vi "Test Remove From Child List.vi"(8 "error in (no error)":errorcluster) -> (0 "error out":errorcluster)   [LabVIEW 2017, in "Unit Tests.lvlib"]
uses:
  Unit Tests.lvlib
  source/Browser Core/Node Classes/Generic Node/Generic Node.lvclass
  source/Browser Core/Node Classes/Generic Node/Generic Node.lvclass/Generic Node.ctl
  <vilib>/addons/_JKI Toolkits/Caraya/classes/Test/Test.lvclass
  <vilib>/addons/_JKI Toolkits/Caraya/classes/Assert/Assert.lvclass
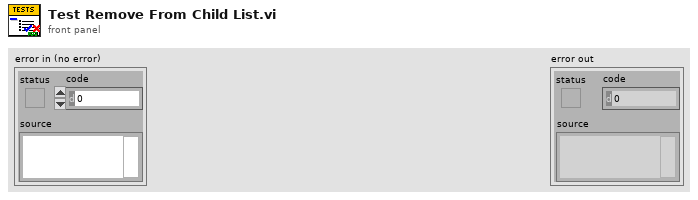
[diagram p1: front panel]
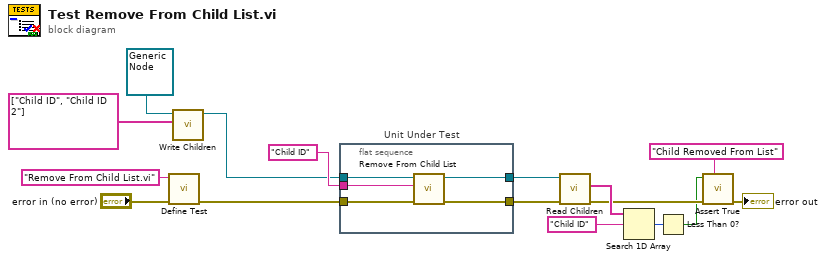
[diagram p0: block diagram]
diagram:
  n1 = call <vilib>:"Define Test.vi"("error in (no error)"="error in (no error)", "Label (VI Title)"="Remove From Child List.vi") -> ("error out"=w10:errorcluster)  [unwired: 9 in]
  n2 = call "Write Children.vi"("Children"=string[] ["Child ID", "Child ID 2"], "Generic Node in"=refnum<class "Generic Node.lvclass"> refnum) -> ("Generic Node out"=w12:refnum<class "Generic Node.lvclass">)  [unwired: 8 in, 1 out]
  n3 = flat-sequence "Unit Under Test" {
    tunnel: w12 -> [w21]
    tunnel: "Child ID" ("Child ID") -> [w20]
    tunnel: w10 -> [w19]
    tunnel: [w18] -> w9
    tunnel: [w17] -> w8
    frame #0 {
      n4 = call "Remove From Child List.vi"("error in (no error)"=w19, "Child ID"=w20, "Generic Node in"=w21) -> ("error out"=w18:errorcluster, "Generic Node out"=w17:refnum<class "Generic Node.lvclass">)  [unwired: 7 in]
    }
  }
  n5 = call "Read Children.vi"("error in (no error)"=w9, "Generic Node in"=w8) -> ("error out"=w4:errorcluster, "Children"=w7:string[])  [unwired: 7 in, 1 out]
  n6 = Search 1D Array(1D array=w7, element="Child ID" ("UID")) -> (index of element=w5:i32)  [unwired: 1 in]
  n7 = Less Than 0?(x=w5) -> (x < 0?=w3:bool)
  n8 = call <vilib>:"Assert True.vi"("Label"="Child Removed From List", "error in (no error)"=w4, "True?"=w3) -> ("error out"=→"error out":errorcluster)  [unwired: 8 in]
